vi "Logger.PGSQL.Write.vi"(8 "error in (no error)":errorcluster, 9 "data in":variant, 10 "address":string, 11 "Logger.PGSQL in":refnum<class "Logger.PGSQL.lvclass">) -> (0 "error out":errorcluster, 2 "Wrote to DB?":bool, 3 "Logger.PGSQL out":refnum<class "Logger.PGSQL.lvclass">)   [LabVIEW 2019, in "Logger.PGSQL.lvlib" / "Logger.PGSQL.lvclass"]
uses:
  Logger.PGSQL.lvclass
  <userlib>/LevyLab/LV-Data/LV-Data.PG/LV-Data.PGSQL.lvclass
  <userlib>/LevyLab/LV-Data/LV-Data.PG/API/Write Variable (one-row).vi
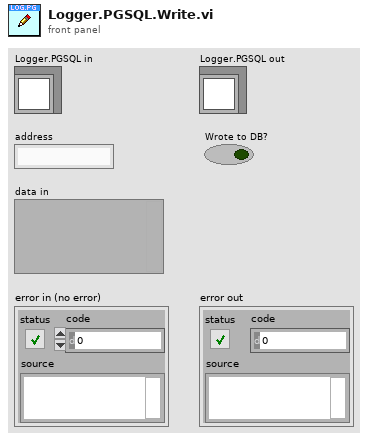
[diagram p1: front panel]
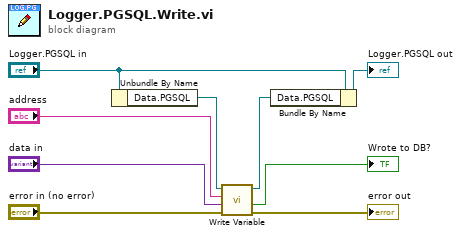
[diagram p0: block diagram]
diagram:
  n1 = Unbundle By Name("Logger.PGSQL in") -> ("Data.PGSQL"=w4:refnum<class "LV-Data.PGSQL.lvclass">)
  n2 = call-poly <userlib>:"Write Variable.vi"("error in (no error)"="error in (no error)", "Data"="data in", "variable"="address", "Data.PG in"=w4) -> ("error out"=→"error out":errorcluster, "Wrote to DB?"=→"Wrote to DB?":bool, "Data.PG out"=w3:refnum<class "LV-Data.PGSQL.lvclass">)  [unwired: 4 in, 1 out]
  n3 = Bundle By Name(cluster="Logger.PGSQL in", "Data.PGSQL"=w3) -> (→"Logger.PGSQL out":refnum<class "Logger.PGSQL.lvclass">)
